vi "计算一组坐标的平均XY.vi"(11 "存储当前铆点的默认位置":cluster{"X":sgl, "Y":sgl}[](array[cluster])) -> (1 "大小":i32, 3 "簇":cluster{"mean":dbl, "mean":dbl})   [LabVIEW 2014]
uses:
  <vilib>/Analysis/baseanly.llb/Mean (DBL).vi
  <vilib>/Analysis/NI_AALBase.lvlib
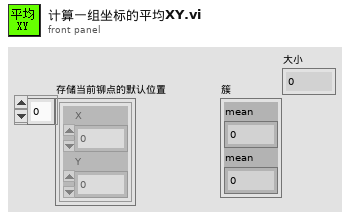
[diagram p1: front panel]
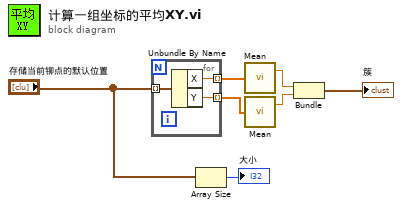
[diagram p0: block diagram]
diagram:
  n1 = for {
    tunnel: "存储当前铆点的默认位置" -> [w10] mode=indexing
    tunnel: [w9] -> w3 mode=indexing
    tunnel: [w8] -> w4 mode=indexing
    n2 = Unbundle By Name(w10) -> ("X"=w9:sgl, "Y"=w8:sgl)
  }
  n3 = Array Size(array="存储当前铆点的默认位置") -> (size(s)=→"大小":i32)
  n4 = call-poly <vilib>:"Mean.vi"("X"=w3) -> ("mean"=w6:dbl)  [unwired: 1 out]
  n5 = call-poly <vilib>:"Mean.vi"("X"=w4) -> ("mean"=w5:dbl)  [unwired: 1 out]
  n6 = Bundle("mean"=w6, "mean"=w5) -> (→"簇":cluster{"mean":dbl, "mean":dbl})  [unwired: 1 in]
